vi "Test Worker Job Count Incremented.vi"(8 "error in (no error)":errorcluster, 11 "Worker Test in":refnum<class "Worker Test.lvclass">) -> (0 "error out":errorcluster, 3 "Worker Test out":refnum<class "Worker Test.lvclass">)   [LabVIEW 2020, in "Worker Test.lvclass"]
uses:
  Worker Test.lvclass
  C:/Program Files (x86)/National Instruments/LabVIEW 2020/vi.lib/Asteme/LUnit/Test Case.lvclass
  <vilib>/Asteme/Triarc Framework/Process/Process.lvclass/Process.ctl
  <vilib>/Asteme/LUnit/Test Case.lvclass/Test Case.ctl
  <vilib>/Asteme/LUnit/LUnit Assertion Result.lvclass/LUnit Assertion Result.ctl
  <vilib>/Asteme/Triarc Framework Test Suite/Support/Execution timer.vi
  <vilib>/Asteme/Triarc Framework/Process/Private/SubVIs/Wait for finish.vi
  <vilib>/Asteme/Triarc Framework/Process/Protected/Messaging/Enqueue Message.vi
  <vilib>/Asteme/Triarc Framework/Process/Private/SubVIs/Set Lifecycle State.vi
  <vilib>/Asteme/Triarc Framework/Process/Public/Lifecycle/Get Lifecycle State.vi
  <vilib>/Asteme/LUnit/Palette/Pass.vi
  <vilib>/Asteme/LUnit/Palette/Fail.vi
  <vilib>/Asteme/LUnit/Variant to string.vi
  <vilib>/Asteme/LUnit/Set Assertion Type.vi
  <vilib>/AdvancedString/1D String Array to Delimited String.vi
  <vilib>/Utility/error.llb/Clear Errors.vi
  <vilib>/Asteme/LUnit/Add test result.vi
  <vilib>/Asteme/LUnit/LUnit Write Passed.vi
  <vilib>/Asteme/LUnit/LUnit Get Test Case.vi
  <vilib>/Asteme/LUnit/Assertion Result/LUnit Get Test Name.vi
  <vilib>/Asteme/LUnit/LUnit Write Message.vi
  <vilib>/Asteme/LUnit/LUnit Write Description.vi
  <vilib>/Asteme/LUnit/LUnit Write Assertion Type.vi
  <vilib>/Asteme/LUnit/Read Test Case Name.vi
  Processes/People/Workers/Worker/Worker.lvclass
  C:/Program Files (x86)/National Instruments/LabVIEW 2020/vi.lib/Asteme/Triarc Framework/Process/Process.lvclass
  <vilib>/Asteme/Triarc Framework Test Suite/Support/Event Helpers/Dequeue Event Message.vi
  <vilib>/Utility/error.llb/Error Cluster From Error Code.vi
  <vilib>/Utility/Data Type/Get Type Information.vi
  <vilib>/Utility/LVClass/Get LV Class Name.vi
  <vilib>/Asteme/LUnit/LUnit Assertion Result.lvclass
  <vilib>/Asteme/Triarc Framework/Process/Process.lvclass
  <vilib>/Asteme/Triarc Framework Test Suite/Support/Event Helpers/Event Helpers.lvlib
  <vilib>/Asteme/LUnit/Test Case.lvclass
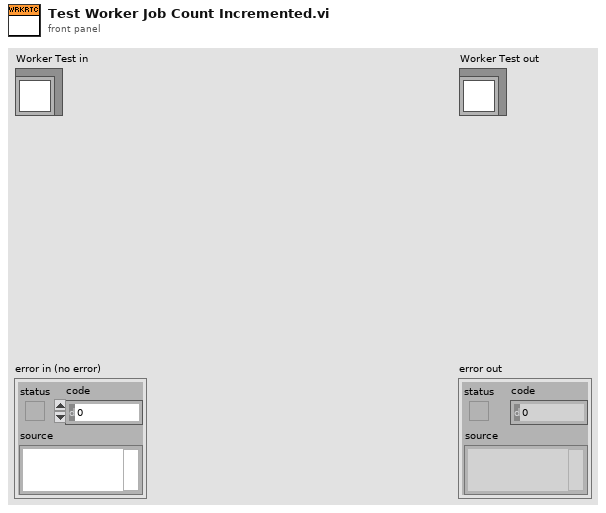
[diagram p1: front panel]
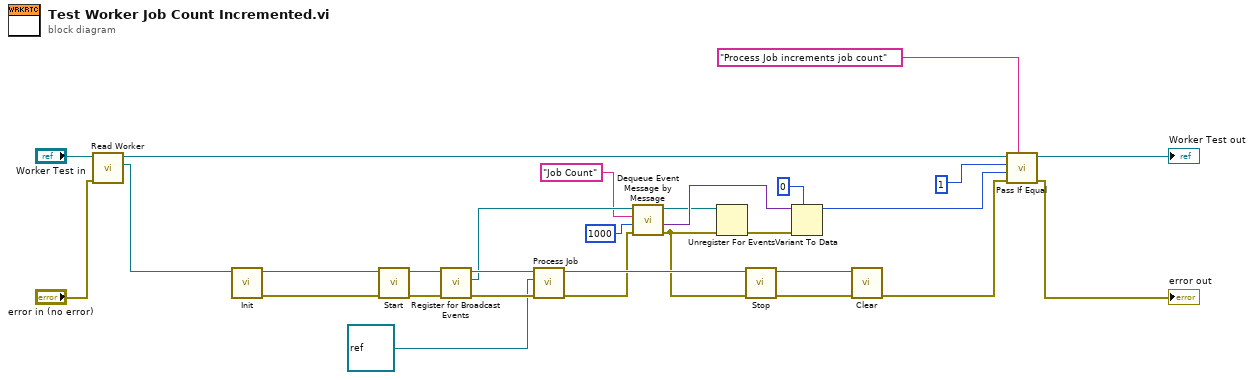
[diagram p0: block diagram]
diagram:
  n1 = call "Read Worker.vi"("error in (no error)"="error in (no error)", "Worker Test in"="Worker Test in") -> ("Worker"=w24:refnum<class "Worker.lvclass">, "Worker Test out"=w26:refnum<class "Worker Test.lvclass">)  [unwired: 7 in, 1 out]
  n2 = call-dynamic "Init.vi"("View In"=w24) -> ("error out"=w23:errorcluster, "View Out"=w20:refnum<class "Worker.lvclass">)  [unwired: 9 in]
  n3 = call <vilib>:"Start.vi"("error in (no error)"=w23, "Process In"=w20) -> ("error out"=w19:errorcluster, "Process Out"=w15:refnum<class "Worker.lvclass">)  [unwired: 8 in]
  n4 = call <vilib>:"Register for Broadcast Events.vi"("error in (no error)"=w19, "Process In"=w15) -> ("error out"=w16:errorcluster, "Event Registration Refnum Out"=w10:refnum<event-registration>, "Process Out"=w14:refnum<class "Worker.lvclass">)  [unwired: 7 in]
  n5 = call-dynamic "Process Job.vi"("error in (no error)"=w16, "Job"=refnum<class> refnum ("Task"), "Worker In"=w14) -> ("error out"=w12:errorcluster, "Worker Out"=w13:refnum<class "Worker.lvclass">)  [unwired: 7 in]
  n6 = call <vilib>:"Dequeue Event Message by Message.vi"("error in (no error)"=w12, "Timeout (-1)"=1000, "Message"="Job Count", "Event Registration Refnum"=w10) -> ("error out"=w4:errorcluster, "Message Data"=w7:variant, "Event Registration Refnum Out"=w1:refnum<event-registration>)  [unwired: 3 in, 2 out]
  n7 = Unregister For Events(event registration refnum=w1, error in=w4) -> (error out=w2:errorcluster)
  n8 = call <vilib>:"Stop.vi"("error in (no error)"=w4, "Process In"=w13) -> ("error out"=w21:errorcluster, "Process Out"=w22:refnum<class "Worker.lvclass">)  [unwired: 7 in, 1 out]
  n9 = Variant To Data(error in=w2, type=u32 0 ("code"), Variant=w7) -> (data=w5:u32)  [unwired: 1 out]
  n10 = call-dynamic "Clear.vi"("error in (no error)"=w21, "View In"=w22) -> ("error out"=w18:errorcluster)  [unwired: 9 in]
  n11 = call <vilib>:"Pass If Equal.vi"("Description"="Process Job increments job count", "error in (no error)"=w18, "Actual"=w5, "Expected"=u32 1 ("code"), "Test Case In"=w26) -> ("error out"=→"error out":errorcluster, "Test Case Out"=→"Worker Test out":refnum<class "Worker Test.lvclass">)  [unwired: 5 in]
